vi "UDP Sender.vi"(4 "error in":errorcluster, 5 "Show panel":bool=TRUE, 6 "boost":dbl=1.0, 7 "Spots":T5={"Spots Settings Array"=[{"x"=10.0, "y"=10.0, "z"=0.0, "Intensity"=0.7000000000000001, "Vortex Charge"=0, "Phase"=0.0}, {"x"=0.0, "y"=0.0, "z"=0.0, "Intensity"=1.0, "Vortex Charge"=0, "Phase"=0.0}], "Current Spot"=2} {"Spots Settings Array"."Phase" step=0.7753; "Spots Settings Array"."Intensity" step=0.1; "Spots Settings Array"."z" step=1e-06; "Spots Settings Array"."y" step=1e-06; "Spots Settings Array"."x" step=1e-06}) -> (0 "error out":errorcluster, 3 "length":i32=234)   [LabVIEW 2014]
doc: "This VI sends UDP packets to the hologram server so that it can display holograms. It also has a lot of settings on the front panel, which control most of the aspects of hologram generation and display."
uses:
  <userlib>/SLM/SLM Spots.ctl
  <vilib>/Analysis/Matrix/Datatypes/RealMatrix.ctl
  <vilib>/Analysis/Matrix/NI_Matrix.lvlib
panel:
  in  "NA Position":cluster{"x":dbl, "y":dbl, "r":dbl}={"x"=0.0, "y"=0.0, "r"=1.0}
  in  "Save settings to defaults file":bool
  in  "SLM Settings":T1(tab)=enum."Aberration"
  in  "Remote Host":string="127.0.0.1"
  in  "Local Port":u16=61556
  in  "Remote Port":u16=61557
  in  "-¹..¹ range control":enum16{"wrap round", "cast to range"}(ring)=enum."cast to range"
  out "'blazing function'":cluster{dbl, dbl}[](graph)=[{-3.141592653589793, 0.0}, {-2.938909256584, 0.05408050907909771}, {-2.736225859578207, 0.10749686306470303}, {-2.533542462572414, 0.1595849068633236}, {-2.330859065566621, 0.20968048538146697}, {-2.1281756685608277, 0.2571194435256408}, {-1.9254922715550344, 0.30123762620235267}, {-1.7228088745492414, 0.3413708783181102}, {-1.5201254775434483, 0.376855044779421}, {-1.317442080537655, 0.40702597049279277}, {-1.114758683531862, 0.43121950036473294}, {-0.9120752865260688, 0.4487714793017492}, {-0.7093918895202758, 0.4591679220820269}, {-0.5067084925144827, 0.4636930977516182}, {-0.3040250955086896, 0.4648168795779257}, {-0.10134169850289654, 0.4650300759565277}, {0.10134169850289654, 0.4668234952830024}, {0.30402509550868917, 0.4726879459529282}, {0.5067084925144831, 0.48479257075013327}, {0.7093918895202758, 0.5033498273826718}, {0.9120752865260693, 0.5278363907764694}, {1.1147586835318615, 0.5577276089708683}, {1.3174420805376554, 0.5924988300052109}, {1.5201254775434485, 0.6316254019188396}, {1.7228088745492416, 0.674582672751097}, {1.9254922715550338, 0.7208459905413253}, {2.1281756685608277, 0.7698907033288669}, {2.330859065566621, 0.8211921591530643}, {2.533542462572414, 0.8742257060532599}, {2.736225859578207, 0.9284666920687961}, {2.938909256584, 0.9833904652390152}, {3.141592653589793, 1.0}]
  in  "Hologram location on-screen":T2={"Display Mode"=0, "Coordinates (x,y,width,height)"=[1920, 0, 512, 512]} {"Display Mode" items=["Coordinates given below", "All of monitor 1", "All of monitor 2", "All of monitor 3", "All of monitor 4", "All of monitor 5"]}
  in  "Aspect Ratio and Centering":T3={"Physical Aspect Ratio (width/height)"=1.0, "Screen Aspect Ratio (width in pixels/height in pixels)"=1.0, "Illumination Centre (range: 0 to 1)"={"x"=0.51, "y"=0.49}} {"Illumination Centre (range: 0 to 1)"."y" min=0.0 max=1.0 step=0.001; "Illumination Centre (range: 0 to 1)"."x" min=0.0 max=1.0 step=0.001}
  in  "Zernike Coefficients":dbl[](array[numeric])=[0.0, 0.0, 0.0, 0.0, 0.0, 0.0, 0.0, 0.0, 0.0, 0.0, 0.0, 0.0]
  in  "Enable":bool
  in  "Multiplier":dbl=1.0
  out "Phase Map":dbl[][](graph)
  in  "Transformation Matrix":T4=[[-1.8560000000000012e-05, -6.3856e-07, 3.10156e-06], [6.385600000000002e-07, -1.8689999999999996e-05, 3.801559999999999e-06], [0.0, 0.0, -4.4699999999999955e-05]]
  out "message":string="<data>\n<spots>\n  -1.919856E-4 -1.805144E-4 0.000000E+0 0.700000 0 0.000000 0.000000 0.000000 1.000000\r\n  0.000000E+0 0.000000E+0 0.000000E+0 1.000000 0 0.000000 0.000000 0.000000 1.000000\r\n\n</spots>\n<totalA>\n1.700000\n</totalA>\n</data>"
  # "Network Settings:\nIn order for this program to display a hologram on the SLM, the SLM server must be running.  Use either the \"hologram_server.exe\" program, or the LabView alternative.  Note that the hologram_server.exe program will only run on relatively recent graphics cards; the LabView version is unsupported, we reccommend all users purchase a recent graphics card (even a relatively inexpensive one) to take advantage of the order-of-magnitude increase in performance.  The port settings should be left as-is (local 61556, remote 61557) and the remote host should be 127.0.0.1 if the server is running on this machine.\n\nIf you are running the server on a different machine, enter the other machine's IP address in the \"remote host\" field.  It's best to have them on the same subnet, preferably connected to the same hub/switch."
  # "Blazing Function\nThis curve controls the output level (0=black, 1=white) for a given phase on the SLM.  It can be used to optimise the hologram to direct as much light as possible into the first diffraction order, and is particularly useful when the SLM has a range of more or less than one wavelength."
  # "Position of SLM Output Window\nThis determines where the hologram image is shown; usually \"all monitor 2\" is the right one, displaying the hologram full-screen on the second monitor.  You can enter coordinates manually if you need finer control.  By default, the hologram generated is square and the output window will be \"letterboxed\", showing solid black on the outside, and having the hologram in the central square (which will fill either the width or the height of the window, whichever is smaller).\n\nFor Hamamatsu SLMs, this is the correct behaviour for all the models we've tested.\nFor Holoeye SLMs, this is also correct, but it does mean you need to be using the centre of the SLM, not the sides.\nFor Boulder SLMs, you may need to use the coordinates to place the window in the top left corner of the SLM screen."
  # "Aspect ratios and Centering\nThe Physical aspect ratio should be the width of the hologram in the real world divided by its height, while the screen aspect ratio refers to its dimensions in pixels.  Most SLMs have square pixels, so these values should both be the same if the whole SLM is to be used.  NB that using a value of 1 is usually correct even if the SLM is non-square, as a square hologram will give more symmetric spots.  It is OK to use a square aspect ratio even if the hologram's size in pixels is not square; the edges of the area will simply be filled in black.\n\nIf the illumination of the SLM is off-centre, moving a spot in Z will also affect its position in X and Y (think of an off-centre lens).  The \"illumination centre\" can correct for this.  Setting this parameter correctly is particularly important if Laguerre-Gauss beams are to be used (i.e. spots with L not equal to 0).  The real centre of the hologram is at 0.5,0.5."
  # "Aberration Correction\nThe engine allows Zernike polynomials to be added to the hologram to compensate for aberrations.  The coefficients can be adjusted here.  The polynomials included are the first 15, ignoring piston and tilt (as these are adjusted for each spot)."
  # "Astig"
  # "Defocus"
  # "Astig"
  # "Tirefoil"
  # "Coma"
  # "Coma"
  # "Tirefoil"
  # "Tirefoil"
  # "Astig"
  # "Spher"
  # "Astig"
  # "Tirefoil"
  # "Scaling Factors\nTo translate between the coordinates used in the rest of the program and the numbers we send to the SLM, it's necessary to scale things.  The control below is a matrix, to allow maximum flexibility when setting up a system- it's useful if, for example, either your SLM or camera is mounted on its side (so x and y are swapped).\n\nMost people can ignore the matrix and just use the 3 diagonal elements for scaling values for X,Y and Z.  Between about 10 and 100 tends to be best (and negative values are sometimes correct)."
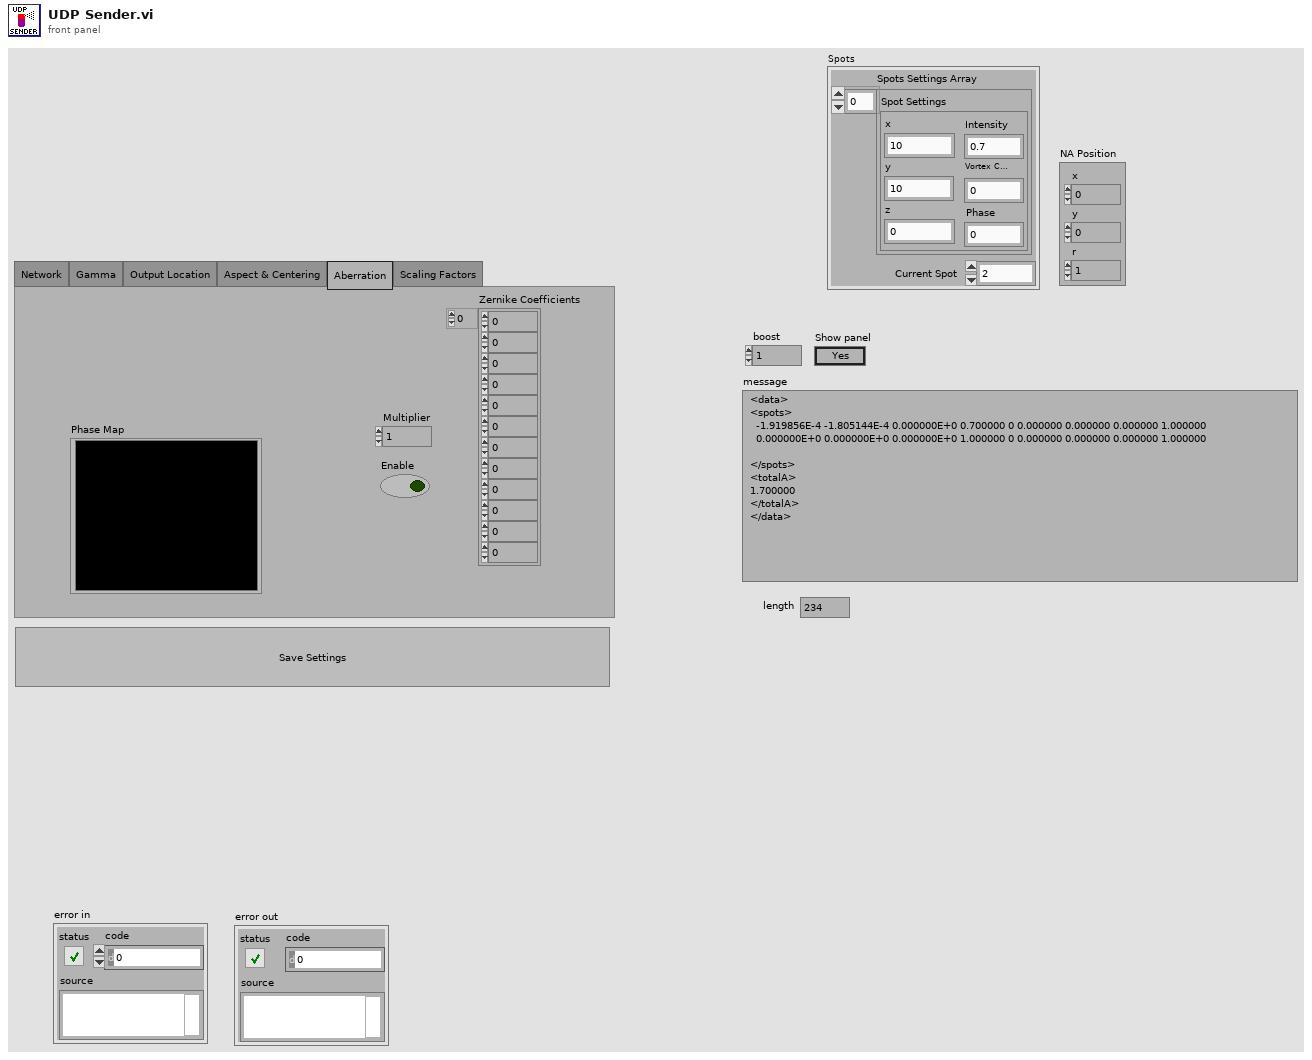
[diagram p1: front panel]
types:
  T1 = enum32{"Network", "Gamma", "Output Location", "Aspect & Centering", "Aberration", "Scaling Factors"}
  T2 = cluster{"Display Mode":u16, "Coordinates (x,y,width,height)":i32[]}
  T3 = cluster{"Physical Aspect Ratio (width/height)":dbl, "Screen Aspect Ratio (width in pixels/height in pixels)":dbl, "Illumination Centre (range: 0 to 1)":cluster{"x":dbl, "y":dbl}}
  T4 = typedef "NI_Matrix.lvlib/RealMatrix.ctl" = dbl[][]
  T5 = typedef "SLM Spots.ctl" = cluster{"Spots Settings Array":cluster{"x":dbl, "y":dbl, "z":dbl, "Intensity":dbl, "Vortex Charge":i8, "Phase":dbl}[], "Current Spot":i32}
  T6 = cluster{"x":dbl, "y":dbl, "z":dbl, "Intensity":dbl, "Vortex Charge":i8, "Phase":dbl}[]
  T7 = typedef "LVCursorListTypeDef.ctl" = cluster{"Name":string, "Color":u32, "Style":u8, "Point Style":u8, "Name Visible":bool, "Allow Drag":bool, "Cursor Mode":u32, "Plot":i32, "Index":i32, "Position":cluster{"X":dbl, "Y":dbl}, "X Scale":u32, "Y Scale":u32, "Watch Plots":i32[], "Watch All Plots":bool, "Plot Area":i32, "Label Offset":cluster{"X":dbl, "Y":dbl}}[]
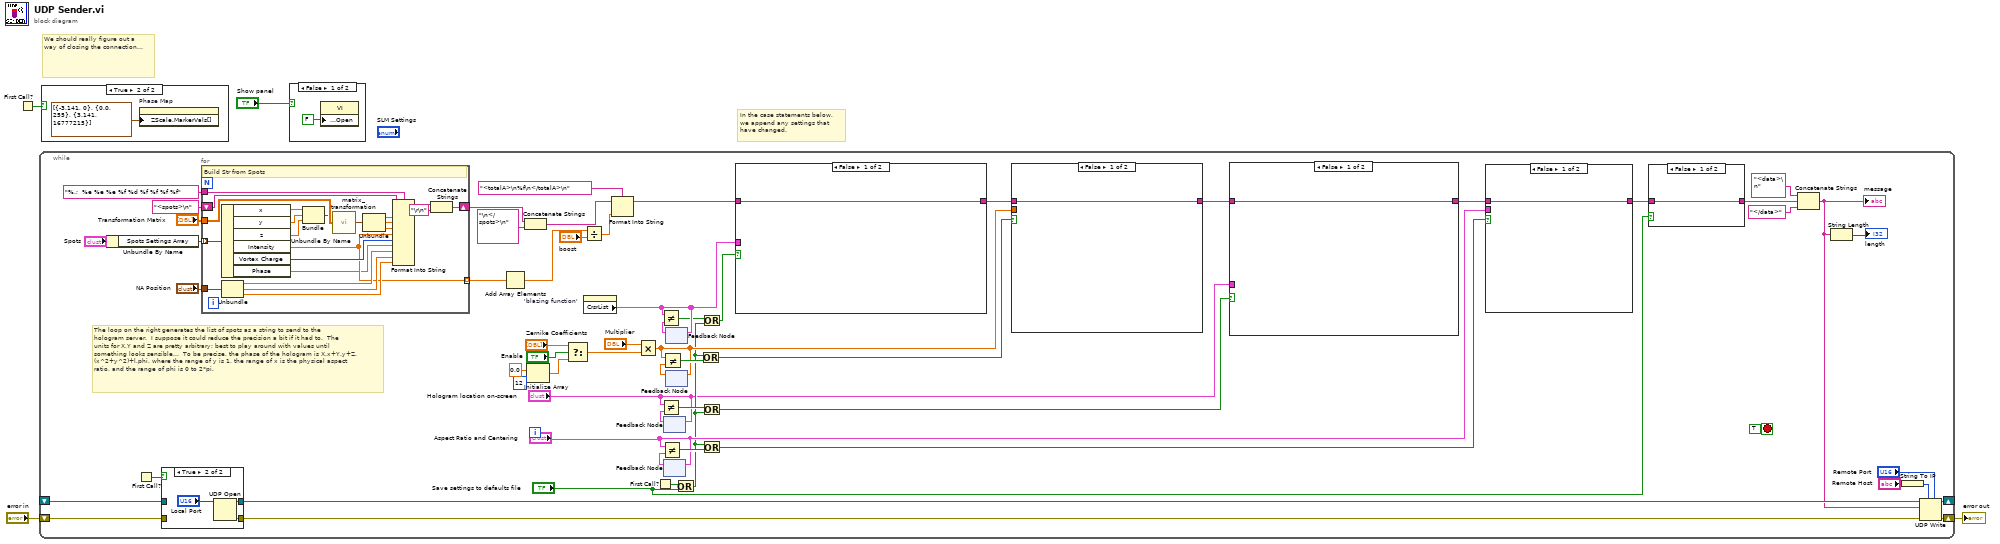
[diagram p0: block diagram]
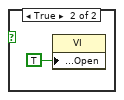
[diagram p3: hidden frame]
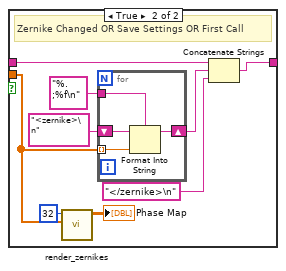
[diagram p4: hidden frame]
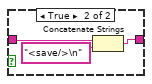
[diagram p5: hidden frame]
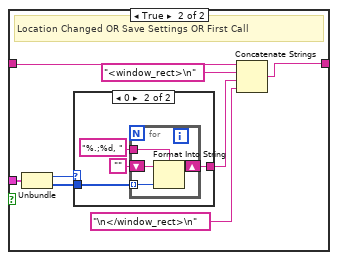
[diagram p6: hidden frame]
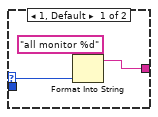
[diagram p7: hidden frame]
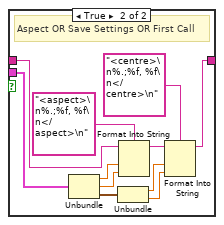
[diagram p8: hidden frame]
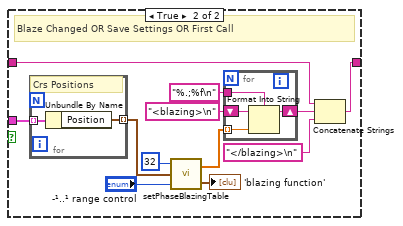
[diagram p9: hidden frame]
diagram:
  # "In the case statements below, we append any settings that have changed."
  # "We should really figure out a way of closing the connection..."
  n1 = First Call?() -> (First Call?: T/F=w3:bool)
  n2 = while {
    shift-right: [w62] -> _
    shift-left: _ -> [w61]
    shift-right: [w63] -> w1
    shift-left: "error in" -> [w60]
    stop <- TRUE stop-if-true
    # "The loop on the right generates the list of spots as a string to send to the hologram server.  I suppose it could reduce the precision a bit if it had to.  The units for X,Y and Z are pretty arbitrary; best to play around with values until something looks sensible...  To be precise, the phase of the hologram is X.x+Y.y+Z.(x^2+y^2)+l.phi, where the range of y is 1, the range of x is the physical aspect ratio, and the range of phi is 0 to 2*pi."
    n3 = Unbundle By Name("Spots") -> ("Spots Settings Array"=w17:T6)
    n4 = First Call?() -> (First Call?: T/F=w41:bool)
    n5 = case shown="True" w41 {
      tunnel: [w158 w160] -> w59
      tunnel: [w157 w159] -> w57
      tunnel: w61 -> [w158 _]
      tunnel: w60 -> [w157 _]
      frame False {
      }
      frame True {
        n6 = UDP Open(11:"Local Port") -> (port=w160:refnum<k16>, 0:w159:errorcluster)  [unwired: 1 in, 4 out]
      }
    }
    n7 = for {
      tunnel: w17 -> [w141] mode=indexing
      shift-right: [w153] -> w56
      shift-left: "<spots>\n" ("Data String") -> [w156]
      tunnel: "%.;  %e %e %e %f %d %f %f %f %f" ("initial string") -> [w155]
      tunnel: "Transformation Matrix" -> [w151]
      tunnel: [w145] -> w32 mode=indexing
      tunnel: "NA Position" -> [w140]
      # "Build Str from Spots"
      n8 = Unbundle By Name(w141) -> ("x"=w138:dbl, "y"=w137:dbl, "z"=w136:dbl, "Intensity"=w145:dbl, "Vortex Charge"=w150:i8, "Phase"=w139:dbl)
      n9 = Unbundle(w140) -> ("x"=w149:dbl, "y"=w148:dbl, "r"=w147:dbl)
      n10 = Bundle("x"=w138, "y"=w137, "z"=w136) -> (w135:cluster{"x":dbl, "y":dbl, "z":dbl})  [unwired: 1 in]
      n11 = call "matrix_transformation.vi"("Transformation Matrix"=w151, "Input Vector"=w135) -> ("Output Vector"=w144:cluster{dbl, dbl, dbl})  [unwired: 1 in, 1 out]
      n12 = Unbundle(w144) -> (w143:dbl, w142:dbl, w152:dbl)
      n13 = Format Into String(format string=w155, initial string=w156, w143, w142, w152, w145, w150, w139, w149, w148, w147) -> (resulting string=w146:string)  [unwired: 1 in, 1 out]
      n14 = Concatenate Strings(w146, "\r\n") -> (w153:string)
    }
    n15 = Add Array Elements(numeric array=w32) -> (sum=w31:dbl)
    n16 = Concatenate Strings(w56, "\n</spots>\n" ("Data String")) -> (w35:string)
    n17 = Initialize Array(0.0 ("element"), 12 ("dimension size")) -> (w25:dbl[])
    n18 = Select(t="Zernike Coefficients", s="Enable", f=w25) -> (s? t:f=w23:dbl[])
    n19 = Divide(x=w31, y="boost") -> (x/y=w34:dbl)
    n20 = property on="'blazing function'" class="XYGraph (strict)"() -> ("CrsrList"=w16:T7)  [unwired: 2 in, 2 out]
    n21 = Format Into String(format string="<totalA>\n%f\n</totalA>\n", initial string=w35, w34) -> (resulting string=w36:string)  [unwired: 1 in, 1 out]
    n22 = Multiply(x="Multiplier", y=w23) -> (x*y=w13:dbl[])
    n23 = First Call?() -> (First Call?: T/F=w14:bool)
    n24 = feedback-in #1("Hologram location on-screen") -> ()
    n25 = feedback #1() -> (w50:T2)  [unwired: 1 out]
    n26 = Not Equal?(x="Hologram location on-screen", y=w50) -> (x != y?=w11:bool)
    n27 = feedback-in #2("Aspect Ratio and Centering") -> ()
    n28 = feedback #2() -> (w45:T3)  [unwired: 1 out]
    n29 = Not Equal?(x="Aspect Ratio and Centering", y=w45) -> (x != y?=w44:bool)
    n30 = feedback-in #3(w16) -> ()
    n31 = feedback #3() -> (w40:T7)  [unwired: 1 out]
    n32 = Not Equal?(x=w16, y=w40) -> (x != y?=w15:bool)
    n33 = feedback-in #4(w13) -> ()
    n34 = feedback #4() -> (w12:dbl[])  [unwired: 1 out]
    n35 = Not Equal?(x=w13, y=w12) -> (x != y?=w28:bool)
    n36 = Or(x=w14, y="Save settings to defaults file") -> (x .or. y?=w10:bool)
    n37 = Or(x=w10, y=w28) -> (x .or. y?=w7:bool)
    n38 = Or(x=w15, y=w10) -> (x .or. y?=w52:bool)
    n39 = Or(x=w11, y=w10) -> (x .or. y?=w48:bool)
    n40 = Or(x=w10, y=w44) -> (x .or. y?=w9:bool)
    n41 = case shown="False" w52 {
      tunnel: w36 -> [w116 w117]
      tunnel: [w116 w125] -> w30
      tunnel: w16 -> [_ w119]
      frame False {
      }
      frame True {
        # "Blaze Changed OR Save Settings OR First Call"
        n42 = for {
          tunnel: w119 -> [w130] mode=indexing
          tunnel: [w129] -> w121 mode=indexing
          # "Crs Positions"
          n43 = Unbundle By Name(w130) -> ("Position"=w129:cluster{"X":dbl, "Y":dbl})
        }
        n44 = call "setPhaseBlazingTable.vi"("-¹..¹ range control"="-¹..¹ range control", "Anchor Points"=w121, "#elements (default 256)"=32) -> ("blazing graph"=→"'blazing function'":cluster{dbl, dbl}[], "blazing table"=w120:dbl[])
        n45 = for {
          shift-right: [w131] -> w126
          shift-left: "<blazing>\n" ("Data String") -> [w134]
          tunnel: "%.;%f\n" ("initial string") -> [w133]
          tunnel: w120 -> [w132] mode=indexing
          n46 = Format Into String(format string=w133, initial string=w134, w132) -> (resulting string=w131:string)  [unwired: 1 in, 1 out]
        }
        n47 = Concatenate Strings(w117, w126, "</blazing>\n" ("Data String")) -> (w125:string)
      }
    }
    n48 = case shown="False" w7 {
      tunnel: w30 -> [w66 w74]
      tunnel: [w66 w73] -> w29
      tunnel: w13 -> [_ w69]
      frame False {
      }
      frame True {
        # "Zernike Changed OR Save Settings OR First Call"
        n49 = call "render_zernikes.vi"("Size"=32, "Coefficients"=w69) -> ("Phase Map"=→"Phase Map":dbl[][])  [unwired: 6 out]
        n50 = for {
          shift-right: [w76] -> w71
          shift-left: "<zernike>\n" -> [w79]
          tunnel: "%.;%f\n" ("initial string") -> [w78]
          tunnel: w69 -> [w77] mode=indexing
          n51 = Format Into String(format string=w78, initial string=w79, w77) -> (resulting string=w76:string)  [unwired: 1 in, 1 out]
        }
        n52 = Concatenate Strings(w74, w71, "</zernike>\n" ("string")) -> (w73:string)
      }
    }
    n53 = case shown="False" w48 {
      tunnel: "Hologram location on-screen" -> [_ w92]
      tunnel: w29 -> [w84 w88]
      tunnel: [w84 w85] -> w47
      frame False {
      }
      frame True {
        # "Location Changed OR Save Settings OR First Call"
        n54 = Unbundle(w92) -> ("Display Mode"=w90:u16, "Coordinates (x,y,width,height)"=w91:i32[])
        n55 = case shown="0" w90 {
          selector: w90 -> [w95 _]
          tunnel: w91 -> [_ w96]
          tunnel: [w93 w97] -> w89
          frame 1, Default {
            n56 = Format Into String(format string="all monitor %d", w95) -> (resulting string=w93:string)  [unwired: 2 in, 1 out]
          }
          frame 0 {
            n57 = for {
              shift-right: [w100] -> w97
              shift-left: "" -> [w103]
              tunnel: "%.;%d, " ("initial string") -> [w102]
              tunnel: w96 -> [w101] mode=indexing
              n58 = Format Into String(format string=w102, initial string=w103, w101) -> (resulting string=w100:string)  [unwired: 1 in, 1 out]
            }
          }
        }
        n59 = Concatenate Strings(w88, "<window_rect>\n" ("Data String"), w89, "\n</window_rect>\n" ("Data String")) -> (w85:string)
      }
    }
    n60 = case shown="False" w9 {
      tunnel: w47 -> [w104 w110]
      tunnel: "Aspect Ratio and Centering" -> [_ w109]
      tunnel: [w104 w105] -> w38
      frame False {
      }
      frame True {
        # "Aspect OR Save Settings OR First Call"
        n61 = Unbundle(w109) -> ("Physical Aspect Ratio (width/height)"=w108:dbl, "Screen Aspect Ratio (width in pixels/height in pixels)"=w107:dbl, "Illumination Centre (range: 0 to 1)"=w106:cluster{"x":dbl, "y":dbl})
        n62 = Unbundle(w106) -> ("x"=w113:dbl, "y"=w112:dbl)
        n63 = Format Into String(format string="<aspect>\n%.;%f, %f\n</aspect>\n", initial string=w110, w108, w107) -> (resulting string=w111:string)  [unwired: 1 in, 1 out]
        n64 = Format Into String(format string="<centre>\n%.;%f, %f\n</centre>\n", initial string=w111, w113, w112) -> (resulting string=w105:string)  [unwired: 1 in, 1 out]
      }
    }
    n65 = case shown="False" "Save settings to defaults file" {
      tunnel: w38 -> [w80 w83]
      tunnel: [w80 w82] -> w42
      frame False {
      }
      frame True {
        n66 = Concatenate Strings(w83, "<save/>\n" ("string")) -> (w82:string)
      }
    }
    n67 = Concatenate Strings("<data>\n" ("Data String"), w42, "</data>" ("Data String")) -> (w20:string)
    "message" <- w20
    n68 = String Length(string=w20) -> (length=→"length":i32)
    n69 = String To IP(1:"Remote Host") -> (0:w51:u32)
    n70 = UDP Write(address=w51, port or service name="Remote Port", connection ID=w59, data in=w20, 8:w57) -> (error out=w63:errorcluster, 3:w62:refnum<k16>)  [unwired: 1 out]
  }
  "error out" <- w1
  n71 = case shown="True" w3 {
    frame False {
    }
    frame True {
      n72 = property on="Phase Map" class="IntGraph (strict)"("ZScale.MarkerVals[]"=cluster{dbl, u32}[] [{-3.141, 0}, {0.0, 255}, {3.141, 16777215}] ("Z Scale.Marker Values[]")) -> ()  [unwired: 2 in, 2 out]
    }
  }
  n73 = case shown="False" "Show panel" {
    frame False {
      n74 = property class="VI"("Front Panel.Open"=FALSE ("Front Panel Window:Open")) -> ()  [unwired: 2 in, 2 out]
    }
    frame True {
      n75 = property class="VI"("Front Panel.Open"=TRUE ("Front Panel Window:Open")) -> ()  [unwired: 2 in, 2 out]
    }
  }
